vi "findTabElement.vi"(8 "error in (no error)":errorcluster, 10 "replaceElementLabeled":string, 11 "Tab ref in":refnum<vi>) -> (0 "error out":errorcluster, 1 "elementReplaced":string, 2 "Tab Control":refnum<vi>, 3 "Tab ref out":refnum<vi>)   [LabVIEW 2011, in "Views.lvlib" / "Camera.lvlib" / "andorSettingsViewer.lvclass"]
uses:
  CameraSettingsViewer/andorSettingsViewer.lvclass
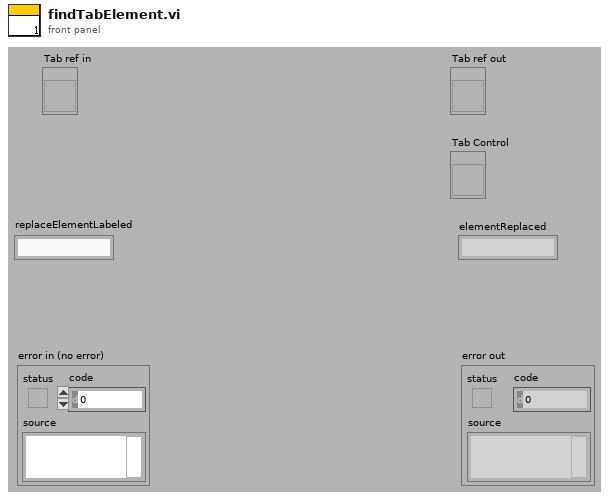
[diagram p1: front panel]
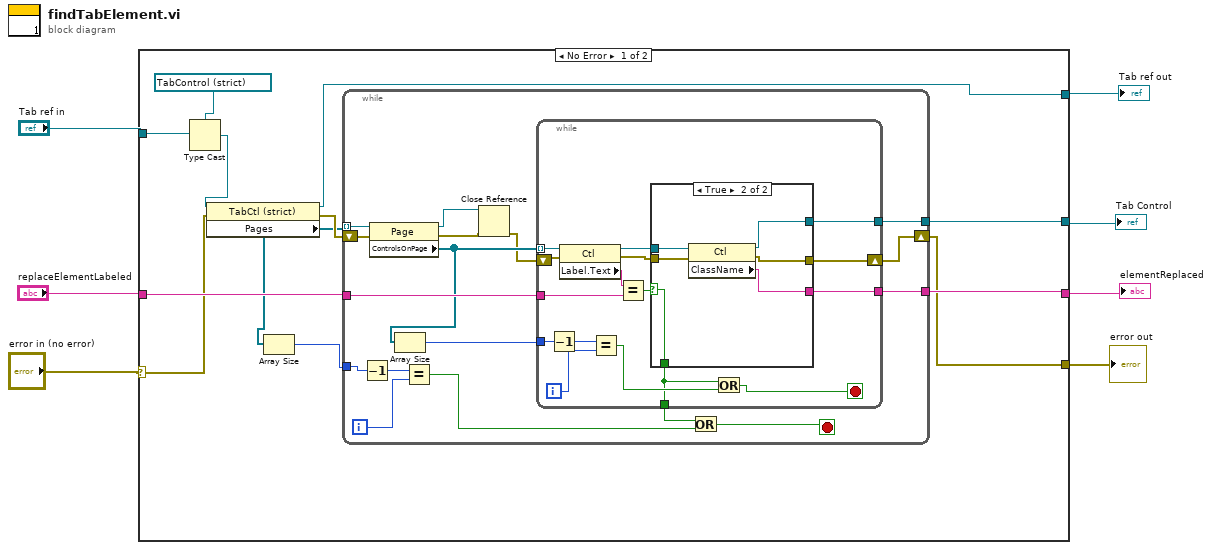
[diagram p0: block diagram]
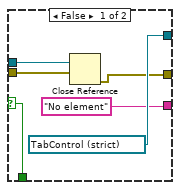
[diagram p2: hidden frame]
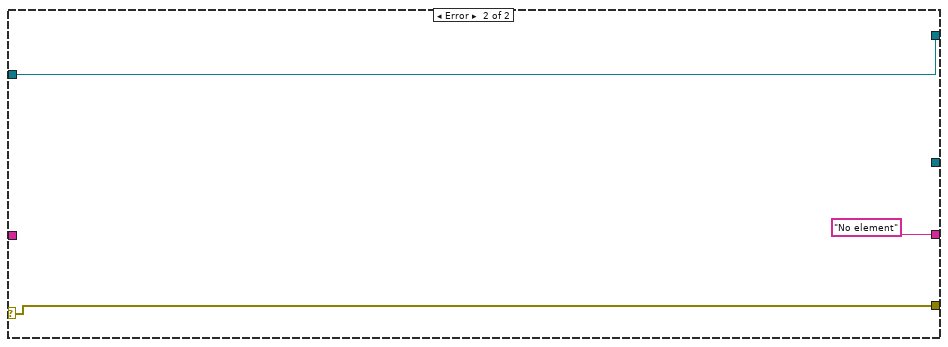
[diagram p3: hidden frame]
diagram:
  n1 = case shown="No Error" "error in (no error)" {
    selector: "error in (no error)" -> [w10 w67]
    tunnel: [w11 w67] -> w6
    tunnel: "Tab ref in" -> [w17 w66]
    tunnel: [w14 w66] -> w4
    tunnel: "replaceElementLabeled" -> [w15 _]
    tunnel: [w13 _] -> w2
    tunnel: [w12 "No element"] -> w1
    frame No Error {
      n2 = Type Cast(type=refnum<vi> refnum ("Tab Control"), x=w17) -> (*(type *) &x=w16:refnum<vi>)
      n3 = property class="TabCtl (strict)"(reference=w16, error in=w10) -> (reference out=w14:refnum<vi>, error out=w19:errorcluster, "Pages"=w9:refnum<vi>[])
      n4 = Array Size(array=w9) -> (size(s)=w8:i32)
      n5 = while {
        tunnel: w9 -> [w36] mode=indexing
        shift-right: [w34] -> w11
        shift-left: w19 -> [w35]
        tunnel: w15 -> [w33]
        tunnel: [w32] -> w13
        tunnel: [w29] -> w12
        tunnel: w8 -> [w27]
        i -> [w26]
        stop <- w23 stop-if-true
        n6 = Decrement(x=w27) -> (x-1=w28:i32)
        n7 = property class="Page"(reference=w36, error in=w35) -> (reference out=w22:refnum<vi>, error out=w21:errorcluster, "ControlsOnPage"=w31:refnum<vi>[])
        n8 = Array Size(array=w31) -> (size(s)=w30:i32)
        n9 = Equal?(x=w28, y=w26) -> (x = y?=w24:bool)
        n10 = Close Reference(reference=w22, error in (no error)=w21) -> (error out=w20:errorcluster)
        n11 = while {
          tunnel: w31 -> [w51] mode=indexing
          tunnel: w33 -> [w50]
          shift-right: [w45] -> w34
          shift-left: w20 -> [w49]
          tunnel: [w44] -> w32
          tunnel: w30 -> [w42]
          tunnel: [w39] -> w29
          tunnel: [w37] -> w25
          i -> [w43]
          stop <- w38 stop-if-true
          n12 = Decrement(x=w42) -> (x-1=w41:i32)
          n13 = property class="Ctl"(reference=w51, error in=w49) -> (reference out=w48:refnum<vi>, error out=w46:errorcluster, "Label.Text"=w52:string)
          n14 = Equal?(x=w41, y=w43) -> (x = y?=w40:bool)
          n15 = Equal?(x=w52, y=w50) -> (x = y?=w47:bool)
          n16 = case shown="True" w47 {
            selector: w47 -> [w53 w59]
            tunnel: w48 -> [w56 w64]
            tunnel: [refnum<vi> refnum ("Tab Control") w63] -> w44
            tunnel: ["No element" w62] -> w39
            tunnel: w46 -> [w55 w61]
            tunnel: [w54 w60] -> w45
            tunnel: [w53 w59] -> w37
            frame False {
              n17 = Close Reference(reference=w56, error in (no error)=w55) -> (error out=w54:errorcluster)
            }
            frame True {
              n18 = property class="Ctl"(reference=w64, error in=w61) -> (reference out=w63:refnum<vi>, error out=w60:errorcluster, "ClassName"=w62:string)
            }
          }
          n19 = Or(x=w37, y=w40) -> (x .or. y?=w38:bool)
        }
        n20 = Or(x=w25, y=w24) -> (x .or. y?=w23:bool)
      }
    }
    frame Error {
    }
  }
  "error out" <- w6
  "Tab ref out" <- w4
  "Tab Control" <- w2
  "elementReplaced" <- w1
